vi "M4_DA_Std_FromBinaryFile.vi"() -> ()   [LabVIEW 2020]
uses:
  spcm_library/spcm_gui_common.llb/element_device.ctl
  spcm_library/spcm_gui_m4i.llb/element_m4i_ao_channel.ctl
  spcm_library/spcm_gui_m4i.llb/element_m4i_ao_trigger.ctl
  spcm_library/spcm_gui_m4i.llb/element_m4i_clock.ctl
  spcm_library/spcm_gui_m4i.llb/element_m4i_multi_purpose_io.ctl
  spcm_library/spcm_gui_common.llb/element_mode_out.ctl
  spcm_library/spcm_gui_common.llb/element_states_replay.ctl
panel:
  in  "Mode Setup":T1={"Mode"=1, "Mem"=4096, "Seg"=1024, "Loop"=0} {"Mode" items=["Singleshot", "Continuous", "Single Restart", "Multiple Replay", "Gated Replay"]; "Loop" step=1; "Mem" min=8 step=4; "Seg" min=8 step=4}
  in  "Multi Purpose IO Lines":T2={"X0 Mode"=0, "ASync Write"=8, "X1 Mode"=0, "X2 Mode"=0} {"X2 Mode" items=["Disable", "Asynchronous In", "Asynchronous Out", "Digital Input (A/D only)", "Digital Output (D/A only)", "Trigger Out", "Digital Input 2Bit (A/D only)", "Show Run State", "Show Arm State", "Ref Clock Out", "Output Marker (D/A only)", "System Clock Out"]; "X1 Mode" items=["Disable", "Asynchronous In", "Asynchronous Out", "Digital Input (A/D only)", "Digital Output (D/A only)", "Trigger Out", "Digital Input 2Bit (A/D only)", "Show Run State", "Show Arm State", "Ref Clock Out", "Output Marker (D/A only)", "System Clock Out"]; "ASync Write" min=8 step=4; "X0 Mode" items=["Disable", "Asynchronous In", "Asynchronous Out", "Digital Input (A/D only)", "Digital Output (D/A only)", "Trigger Out", "Digital Input 2Bit (A/D only)", "Show Run State", "Show Arm State", "Ref Clock Out", "Output Marker (D/A only)", "System Clock Out"]}
  in  "Clock Settings":T3={"Clock Mode"=0, "Sampling Rate (MHz)"=1250.0, "Reference Clock (MHz)"=1000.0, "Clock Output"=FALSE} {"Clock Mode" items=["Internal Clock Quartz", "External Clock (Reference Clock)", "Quartz 2 with PLL (Optional)"]; "Reference Clock (MHz)" min=10.0 max=125000.0; "Sampling Rate (MHz)" min=1.0 max=200000.0}
  in  "Reload data":bool
  out "Data Transfer Progress":i32(slide)=6 scale=0.0..100.0 scale format="%.0f %%"
  out "Replay Started":bool
  out "Data Transferred":bool
  in  "Start Data Transfer":bool
  in  "Ch3":string="waveforms\\rectangle.bin"
  in  "Ch2 File":string="waveforms\\sine.bin"
  in  "Ch1 File":string="waveforms\\Sin96.bin"
  in  "Ch0 File":string="waveforms\\Sin95.bin"
  out "Status":string="Stopped"
  in  "Trigger Settings":T4 {"Secondary Ext. Trigger" items=["None", "Pos. Edge", "Neg. Edge", "Any Edge", "High Level", "Low Level"]; "AC Coupling" items=["DC Coupling", "AC Coupling"]; "Main Ext. Trigger" items=["None", "Pos. Edge", "Neg. Edge", "Any Edge", "Pos. Rearm", "Neg. Rearm", "Enter Window", "Leave Window", "High Level", "Low Level", "In Win", "Out Win", ""]; "Trigger Source" items=["Software Trigger", "Main External Trigger", "Secondary External Trigger"]; "Trigger Delay (Samples)" max=65535 step=1}
  in  "Stop Level":cluster{"Stoplevel":u16}={"Stoplevel"=4} {"Stoplevel" items=["Tristate", "Low Level", "High Level", "Hold Last Sample", "Zero"]}
  in  "Output Channel 3":T5={"Enable"=FALSE, "Output Mode"=0, "Gain"=2000, "Offset"=0, "Filter"=0} {"Output Mode" items=["Single", "Double", "Differential"]}
  in  "Output Channel 2":T5={"Enable"=TRUE, "Output Mode"=0, "Gain"=2000, "Offset"=0, "Filter"=0} {"Output Mode" items=["Single", "Double", "Differential"]}
  in  "Output Channel 1":T5={"Enable"=FALSE, "Output Mode"=0, "Gain"=550, "Offset"=0, "Filter"=0} {"Output Mode" items=["Single", "Double", "Differential"]}
  in  "Output Channel 0":T5={"Enable"=TRUE, "Output Mode"=0, "Gain"=550, "Offset"=0, "Filter"=0} {"Output Mode" items=["Single", "Double", "Differential"]}
  in  "Singleshot Button":bool
  out "Write Setup":bool
  in  "Quit Button":bool
  in  "Force Trigger Button":bool
  in  "Stop Button":bool
  out "Device Infos":T6={"Device Name"="M4i.6622-Exp", "Serial Number"=66.0, "Mem (MB)"=4096.0}
  in  "Device":T7 {"Device" items=["Card", "digitizerNETBOX"]}
  # "Ch1"
  # "Ch0"
  # "Ch3"
  # "Ch2"
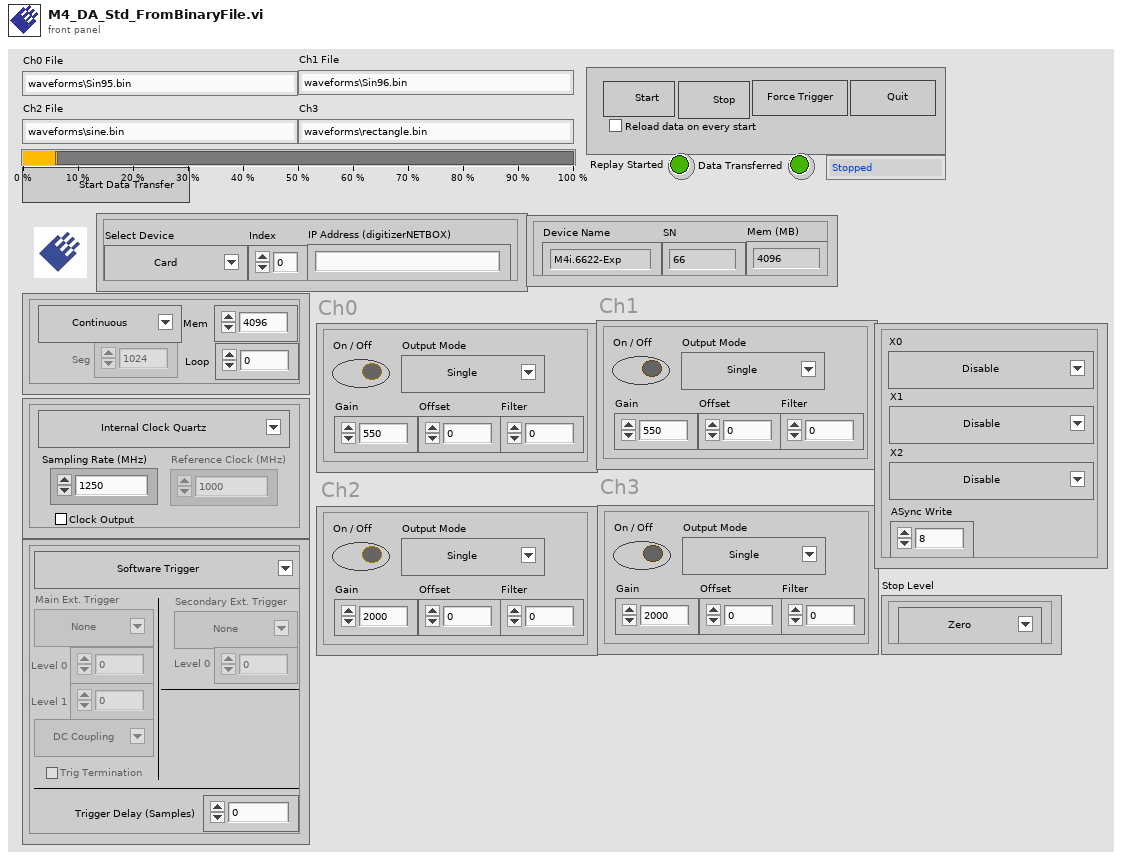
[diagram p1: front panel]
types:
  T1 = typedef "element_mode_out.ctl" = cluster{"Mode":u16, "Mem":u32, "Seg":u32, "Loop":u32}
  T2 = typedef "element_m4i_multi_purpose_io.ctl" = cluster{"X0 Mode":u16, "ASync Write":u32, "X1 Mode":u16, "X2 Mode":u16}
  T3 = typedef "element_m4i_clock.ctl" = cluster{"Clock Mode":u16, "Sampling Rate (MHz)":dbl, "Reference Clock (MHz)":dbl, "Clock Output":bool}
  T4 = typedef "element_m4i_ao_trigger.ctl" = cluster{"Trigger Source":u16, "Main Ext. Trigger":u16, "Level 0 Ext":i32, "Level 1 Ext":i32, "AC Coupling":u16, "Ext Trig Term":bool, "Secondary Ext. Trigger":u16, "Level 0 Ext1":i32, "Trigger Delay (Samples)":u32}
  T5 = typedef "element_m4i_ao_channel.ctl" = cluster{"Enable":bool, "Output Mode":u16, "Gain":i32, "Offset":i32, "Filter":i32}
  T6 = cluster{"Device Name":string, "Serial Number":dbl, "Mem (MB)":dbl}
  T7 = typedef "element_device.ctl" = cluster{"Index":dbl, "IP Address":string, "Device":u16}
  T8 = typedef "element_states_replay.ctl" = enum16{"Idle", "Init", "Write Setup", "Write Data", "Start", "Replay", "Stop", "Quit"}
  T9 = cluster{"Card Type":i32, "Inst Mem (high part)":i32, "Inst Mem (low part)":i32, "Serial Number":i32, "Function Type":i32, "Installed Features":i32, "Base Card Version":i32, "Module Version":i32, "Extension Version":i32, "Production Date":i32, "Max Sampling Rate":i32, "Max Channels":i32, "Demo Card":i32}
  T10 = cluster{"Card Name":string, "SN":i32, "Mem (MB)":i32}
  T11 = cluster{"AO Channels":i32, "Bit Resolution":i32, "AO Gain":i32, "AO Filter":i32, "AO Offset":i32}
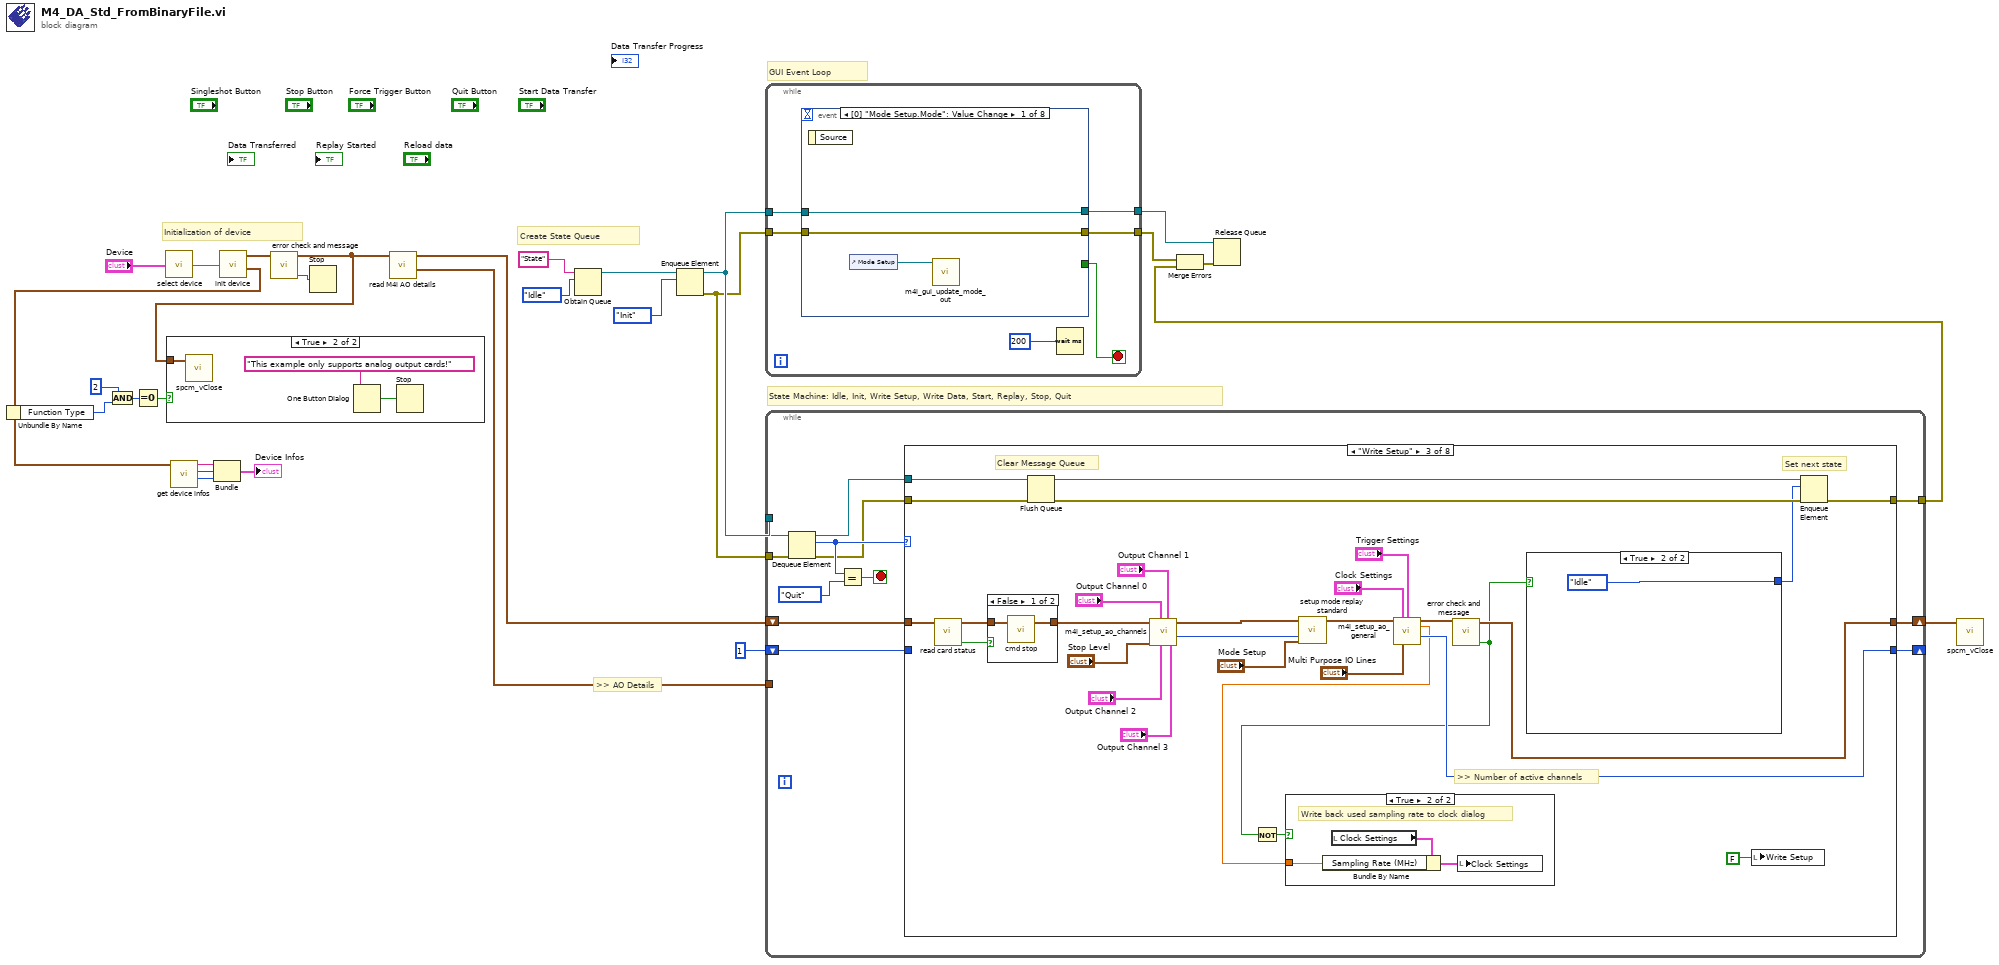
[diagram p0: block diagram]
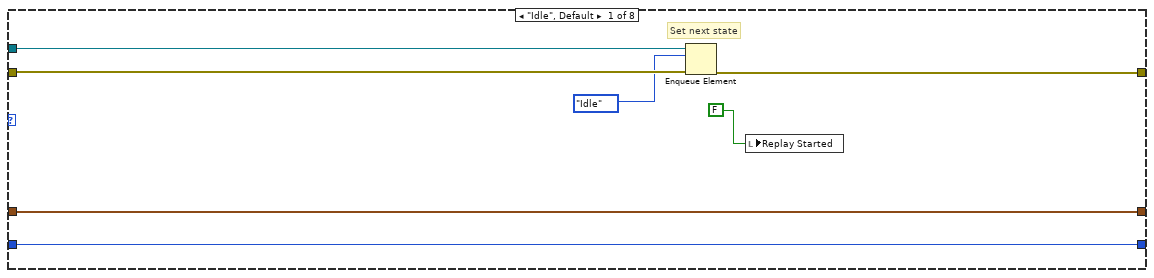
[diagram p3: hidden frame]
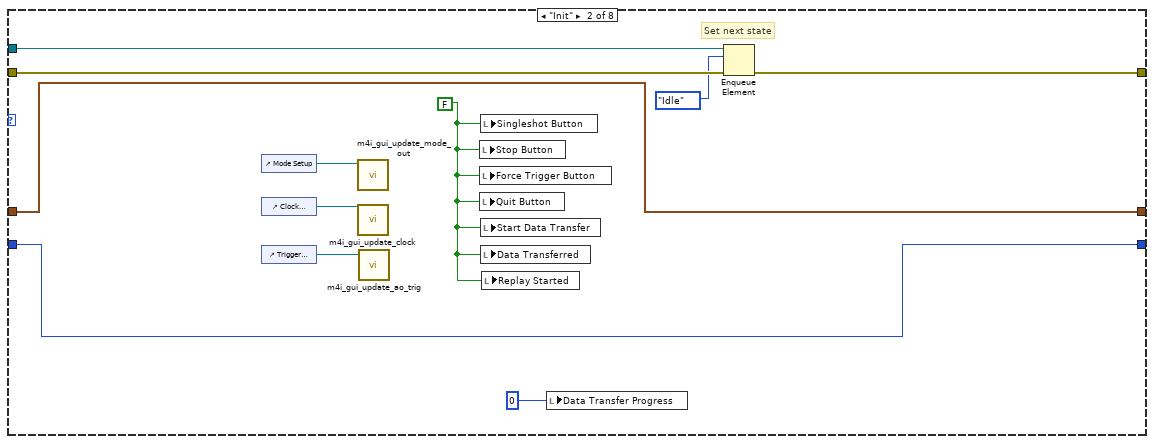
[diagram p4: hidden frame]
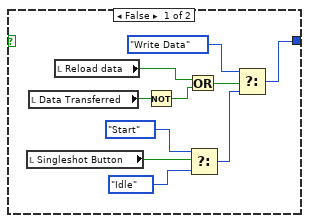
[diagram p7: hidden frame]
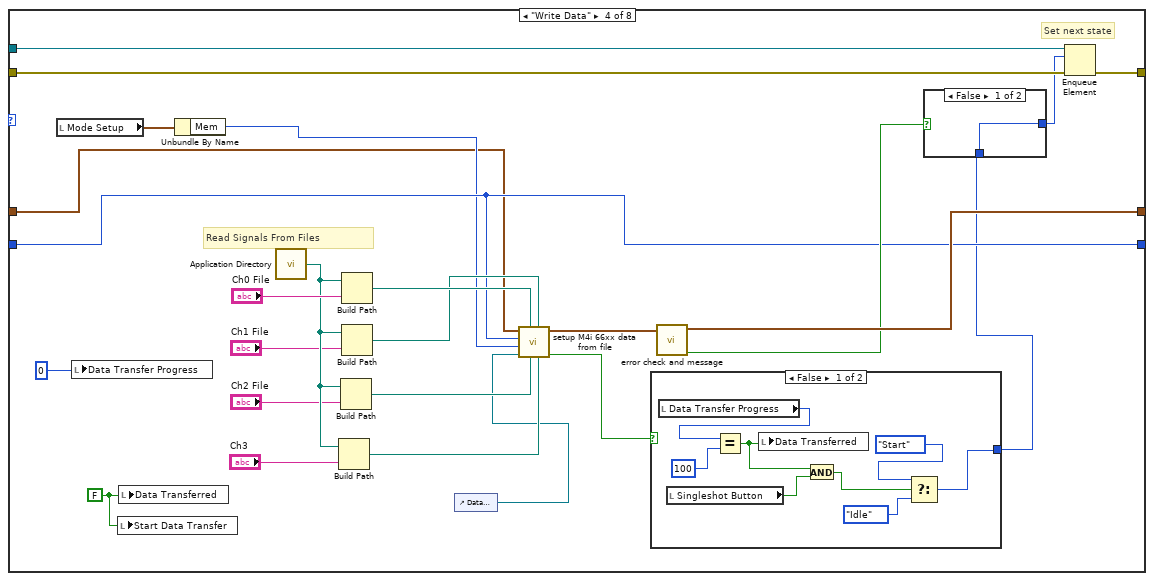
[diagram p8: hidden frame]
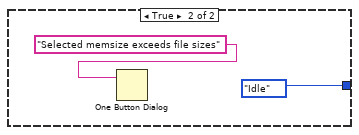
[diagram p9: hidden frame]
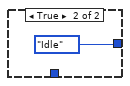
[diagram p10: hidden frame]
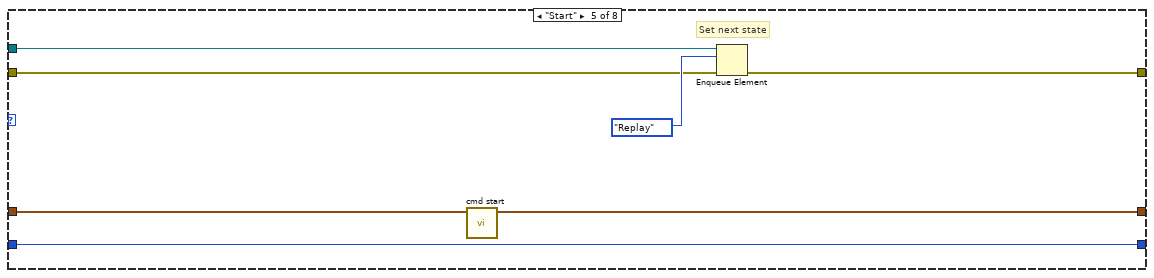
[diagram p11: hidden frame]
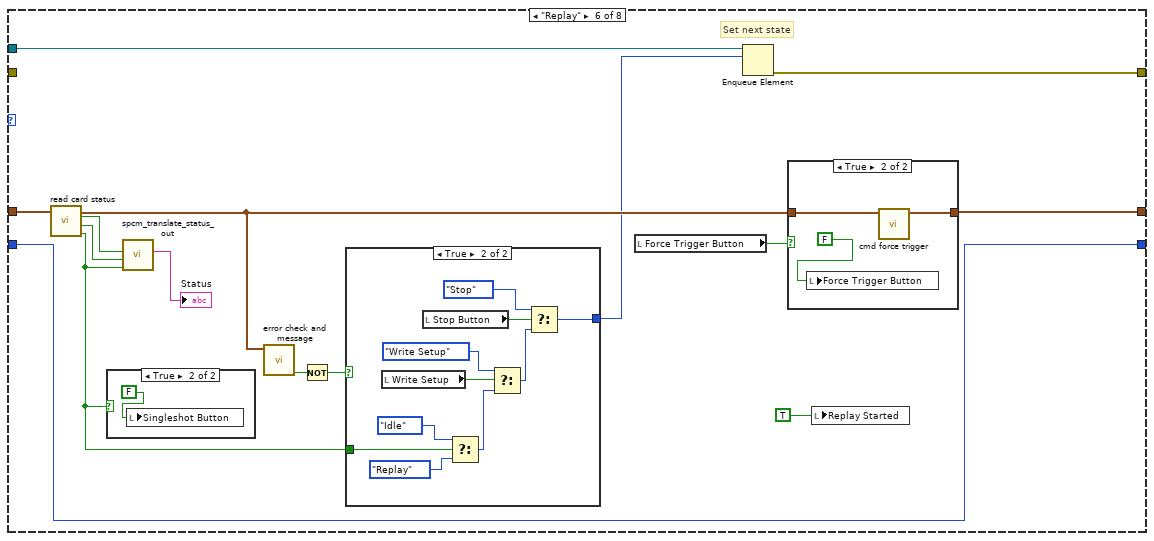
[diagram p12: hidden frame]
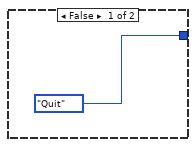
[diagram p14: hidden frame]
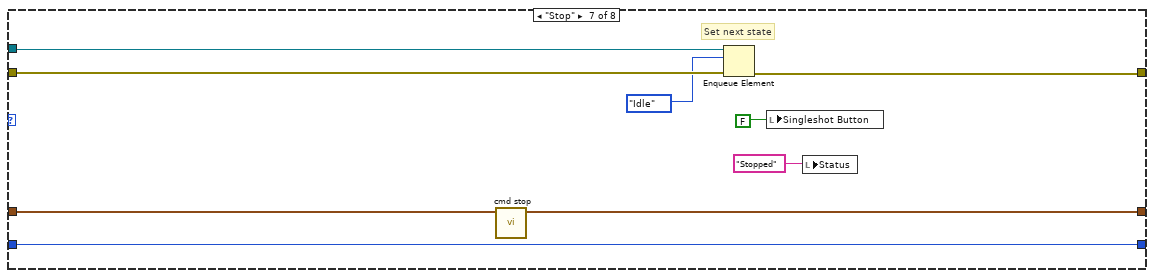
[diagram p16: hidden frame]
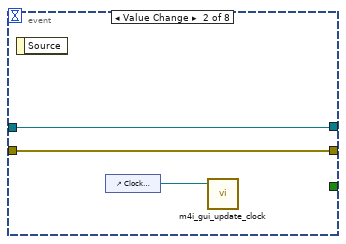
[diagram p18: hidden frame]
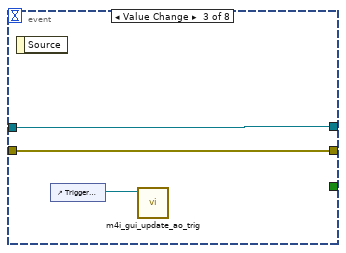
[diagram p19: hidden frame]
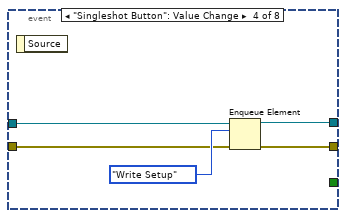
[diagram p20: hidden frame]
diagram:
  # ">> AO Details"
  # "Initialization of device"
  # "Create State Queue"
  # "State Machine: Idle, Init, Write Setup, Write Data, Start, Replay, Stop, Quit"
  # "GUI Event Loop"
  n1 = call "select device.vi"("Device"="Device") -> ("device string"=w28:string)  [unwired: 4 in]
  n2 = call "init device.vi"("Device String"=w28) -> ("Card Info Out"=w27:cluster{"Card Handle":u64, "Error Code":u32}, "Card Information"=w11:T9)  [unwired: 4 in]
  n3 = Unbundle By Name(w11) -> ("Function Type"=w15:i32)
  n4 = And(x=2, y=w15) -> (x .and. y?=w14:i32)
  n5 = Equal To 0?(x=w14) -> (x = 0?=w12:bool)
  n6 = call "get device infos.vi"("Card Information"=w11) -> ("Mem (MB)"=w19:i32, "SN"=w18:i32, "Card Name"=w17:string)  [unwired: 8 in]
  n7 = Bundle("Card Name"=w17, "SN"=w18, "Mem (MB)"=w19) -> (→"Device Infos":T10)  [unwired: 1 in]
  n8 = call "error check and message.vi"("Card Info In"=w27) -> ("Error occurred"=w26:bool, "Card Info Out"=w4:cluster{"Card Handle":u64, "Error Code":u32})  [unwired: 4 in, 1 out]
  n9 = case shown="True" w12 {
    tunnel: w4 -> [_ w29]
    frame False {
    }
    frame True {
      n10 = call "spcm_vClose.vi"("Card Info In"=w29) -> ()  [unwired: 7 in]
      n11 = One Button Dialog(message="This example only supports analog output cards!") -> (true=w30:bool)  [unwired: 1 in]
      n12 = Stop(stop? (T)=w30) -> ()
    }
  }
  n13 = Stop(stop? (T)=w26) -> ()
  n14 = call "read M4i AO details.vi"("Card Info In"=w4) -> ("AO Details"=w3:T11, "Card Info Out"=w2:cluster{"Card Handle":u64, "Error Code":u32})  [unwired: 5 in]
  n15 = Obtain Queue(name (unnamed)="State", element data type=element_states_replay."Idle") -> (queue out=w23:refnum<queue>)  [unwired: 3 in, 2 out]
  n16 = Enqueue Element(queue=w23, element=element_states_replay."Init") -> (queue out=w24:refnum<queue>, error out=w6:errorcluster)  [unwired: 2 in, 1 out]
  n17 = while {
    tunnel: w24 -> [w35]
    tunnel: [w36] -> w7
    tunnel: [w32] -> w10
    tunnel: w6 -> [w33]
    stop <- w34 stop-if-true
    n18 = event shown="[0] \"Mode Setup.Mode\": Value Change" {
      selector: _ -> [_ _ _ _ _ _ _ _]
      dyn-events: _ -> [_ _ _ _ _ _ _ _]
      timeout: _ -> [_ _ _ _ _ _ _ _]
      tunnel: [_ _ _ _ _ _ TRUE _] -> w34
      tunnel: [w40 w43 w46 w51 w56 w62 w67 w71] -> w36
      tunnel: w35 -> [w40 w43 w46 w48 w55 w61 w68 w71]
      tunnel: [w39 w42 w45 w50 w53 w59 w65 w70] -> w32
      tunnel: w33 -> [w39 w42 w45 w47 w54 w60 w64 w70]
      event Value Change {
        n19 = event-data ("Ereignisdatenknoten")() -> ()  [unwired: 1 in, 1 out]
        n20 = control-ref of="Mode Setup"() -> (w38:refnum<vi>)
        n21 = call "m4i_gui_update_mode_out.vi"("Cluster Referenz"=w38) -> ()  [unwired: 11 in]
      }
      event Value Change {
        n22 = event-data() -> ()  [unwired: 1 in, 1 out]
        n23 = control-ref of="Clock Settings"() -> (w41:refnum<vi>)
        n24 = call "m4i_gui_update_clock.vi"("Cluster Reference"=w41) -> ()  [unwired: 11 in]
      }
      event Value Change {
        n25 = event-data() -> ()  [unwired: 1 in, 1 out]
        n26 = control-ref of="Trigger Settings"() -> (w44:refnum<vi>)
        n27 = call "m4i_gui_update_ao_trig.vi"("Cluster Referenz"=w44) -> ()  [unwired: 11 in]
      }
      event "Singleshot Button": Value Change {
        n28 = event-data() -> ()  [unwired: 1 in, 1 out]
        n29 = Enqueue Element(queue=w48, element=element_states_replay."Write Setup", error in (no error)=w47) -> (queue out=w51:refnum<queue>, error out=w50:errorcluster)  [unwired: 1 in, 1 out]
      }
      event "Stop Button": Value Change {
        n30 = event-data() -> ()  [unwired: 1 in, 1 out]
        n31 = Enqueue Element(queue=w55, element=element_states_replay."Stop", error in (no error)=w54) -> (queue out=w56:refnum<queue>, error out=w53:errorcluster)  [unwired: 1 in, 1 out]
      }
      event "Start Data Transfer": Value Change {
        n32 = event-data() -> ()  [unwired: 1 in, 1 out]
        n33 = local write "Data Transferred"(FALSE) -> ()
        n34 = Enqueue Element(queue=w61, element=element_states_replay."Write Setup", error in (no error)=w60) -> (queue out=w62:refnum<queue>, error out=w59:errorcluster)  [unwired: 1 in, 1 out]
      }
      event "Quit Button": Value Change {
        n35 = event-data() -> ()  [unwired: 1 in, 1 out]
        n36 = Enqueue Element(queue=w68, element=element_states_replay."Quit", error in (no error)=w64) -> (queue out=w67:refnum<queue>, error out=w65:errorcluster)  [unwired: 1 in, 1 out]
      }
      event Value Change {
        n37 = event-data() -> ()  [unwired: 1 in, 1 out]
        "Write Setup" <- TRUE
      }
    }
    n38 = Wait (ms)(milliseconds to wait=200) -> ()  [unwired: 1 out]
  }
  n39 = while {
    tunnel: w24 -> [w83]
    shift-right: [w81] -> w22
    shift-left: w2 -> [w82]
    shift-right: [w76] -> _
    shift-left: 1 -> [w77]
    tunnel: [w75] -> w9
    tunnel: w6 -> [w74]
    tunnel: w3 -> [_]
    stop <- w79 stop-if-true
    n40 = Dequeue Element(queue=w83, error in (no error)=w74) -> (queue out=w78:refnum<queue>, element=w80:T8, error out=w73:errorcluster)  [unwired: 1 in, 1 out]
    n41 = Equal?(x=w80, y=element_states_replay."Quit") -> (x = y?=w79:bool)
    n42 = case shown="\"Write Setup\"" w80 {
      tunnel: w82 -> [w90 w98 w115 w154 w187 w203 w227 w233]
      tunnel: [w90 w98 w111 w168 w186 w196 w226 w233] -> w81
      tunnel: w78 -> [w85 w101 w117 w170 w185 w199 w230 _]
      tunnel: w77 -> [w89 w97 _ w156 w190 w194 w225 w232]
      tunnel: [w89 w97 w125 w156 w190 w194 w225 w232] -> w76
      tunnel: [w87 w100 w128 w169 w189 w197 w228 w231] -> w75
      tunnel: w73 -> [w88 w99 w129 w171 w184 _ w229 w231]
      frame "Idle", Default {
        # "Set next state"
        n43 = Enqueue Element(queue=w85, element=element_states_replay."Idle", error in (no error)=w88) -> (error out=w87:errorcluster)  [unwired: 1 in, 2 out]
        n44 = local write "Replay Started"(FALSE) -> ()
      }
      frame "Init" {
        w94 = FALSE
        # "Set next state"
        n45 = control-ref of="Mode Setup"() -> (w91:refnum<vi>)
        n46 = control-ref of="Clock Settings"() -> (w92:refnum<vi>)
        n47 = control-ref of="Trigger Settings"() -> (w95:refnum<vi>)
        n48 = call "m4i_gui_update_mode_out.vi"("Cluster Referenz"=w91) -> ()  [unwired: 11 in]
        n49 = call "m4i_gui_update_clock.vi"("Cluster Reference"=w92) -> ()  [unwired: 11 in]
        n50 = call "m4i_gui_update_ao_trig.vi"("Cluster Referenz"=w95) -> ()  [unwired: 11 in]
        n51 = local write "Stop Button"(w94) -> ()
        n52 = local write "Force Trigger Button"(w94) -> ()
        n53 = local write "Quit Button"(w94) -> ()
        n54 = local write "Singleshot Button"(w94) -> ()
        n55 = local write "Start Data Transfer"(w94) -> ()
        n56 = local write "Data Transferred"(w94) -> ()
        n57 = local write "Replay Started"(w94) -> ()
        n58 = local write "Data Transfer Progress"(0) -> ()
        n59 = Enqueue Element(queue=w101, element=element_states_replay."Idle", error in (no error)=w99) -> (error out=w100:errorcluster)  [unwired: 1 in, 2 out]
      }
      frame "Write Setup" {
        # "Set next state"
        # "Clear Message Queue"
        # ">> Number of active channels"
        n60 = call "read card status.vi"("Card Info In"=w115) -> ("Card ready"=w112:bool, "Card Info Out"=w114:cluster{"Card Handle":u64, "Error Code":u32})  [unwired: 3 in, 2 out]
        n61 = case shown="False" w112 {
          tunnel: w114 -> [w134 w135]
          tunnel: [w133 w135] -> w113
          frame False {
            n62 = call "cmd stop.vi"("Card Info In"=w134) -> ("Card Info Out"=w133:cluster{"Card Handle":u64, "Error Code":u32})  [unwired: 6 in]
          }
          frame True {
          }
        }
        n63 = Flush Queue(queue=w117) -> (queue out=w116:refnum<queue>)  [unwired: 1 in, 2 out]
        n64 = call "m4i_setup_ao_channels.vi"("Output Channel 3"="Output Channel 3", "Output Channel 1"="Output Channel 1", "Output Channel 2"="Output Channel 2", "Output Channel 0"="Output Channel 0", "Stop Level"="Stop Level", "Card Info In"=w113) -> ("ChMask"=w103:i32, "Card Info Out"=w104:cluster{"Card Handle":u64, "Error Code":u32})  [unwired: 3 in, 1 out]
        n65 = call "setup mode replay standard.vi"("Mode Setup"="Mode Setup", "Channel Mask Low"=w103, "Card Info In"=w104) -> ("Card Info Out"=w105:cluster{"Card Handle":u64, "Error Code":u32})  [unwired: 4 in]
        n66 = call "m4i_setup_ao_general.vi"("Card Info In"=w105, "Clock Settings"="Clock Settings", "Trigger Settings"="Trigger Settings", "Multi Purpose IO Lines"="Multi Purpose IO Lines") -> ("Card Info Out"=w118:cluster{"Card Handle":u64, "Error Code":u32}, "Used Sampling Rate (MS)"=w109:dbl, "Channel Count"=w125:i32)  [unwired: 7 in, 2 out]
        n67 = call "error check and message.vi"("Card Info In"=w118) -> ("Error occurred"=w106:bool, "Card Info Out"=w111:cluster{"Card Handle":u64, "Error Code":u32})  [unwired: 4 in, 1 out]
        n68 = Not(x=w106) -> (.not. x?=w107:bool)
        n69 = case shown="True" w107 {
          tunnel: w109 -> [_ w130]
          frame False {
          }
          frame True {
            # "Write back used sampling rate to clock dialog"
            n70 = local read "Clock Settings"() -> (w132:T3)
            n71 = Bundle By Name(cluster=w132, "Sampling Rate (MHz)"=w130) -> (w131:T3)
            n72 = local write "Clock Settings"(w131) -> ()
          }
        }
        n73 = case shown="True" w106 {
          tunnel: [w140 element_states_replay."Idle"] -> w127
          frame False {
            n74 = local read "Singleshot Button"() -> (w137:bool)
            n75 = local read "Data Transferred"() -> (w141:bool)
            n76 = local read "Reload data"() -> (w143:bool)
            n77 = Not(x=w141) -> (.not. x?=w142:bool)
            n78 = Or(x=w143, y=w142) -> (x .or. y?=w144:bool)
            n79 = Select(t=element_states_replay."Start", s=w137, f=element_states_replay."Idle") -> (s? t:f=w136:T8)
            n80 = Select(t=element_states_replay."Write Data", s=w144, f=w136) -> (s? t:f=w140:T8)
          }
          frame True {
          }
        }
        n81 = local write "Write Setup"(FALSE) -> ()
        n82 = Enqueue Element(queue=w116, element=w127, error in (no error)=w129) -> (error out=w128:errorcluster)  [unwired: 1 in, 2 out]
      }
      frame "Write Data" {
        w148 = FALSE
        # "Read Signals From Files"
        # "Set next state"
        n83 = local read "Mode Setup"() -> (w147:T1)
        n84 = local write "Data Transfer Progress"(0) -> ()
        n85 = local write "Start Data Transfer"(w148) -> ()
        n86 = local write "Data Transferred"(w148) -> ()
        n87 = Unbundle By Name(w147) -> ("Mem"=w155:u32)
        n88 = call <vilib>:"Application Directory.vi"() -> ("Application Directory"=w164:path)
        n89 = Build Path(base path=w164, name or relative path="Ch3") -> (appended path=w157:path)
        n90 = Build Path(base path=w164, name or relative path="Ch2 File") -> (appended path=w158:path)
        n91 = Build Path(base path=w164, name or relative path="Ch0 File") -> (appended path=w160:path)
        n92 = Build Path(base path=w164, name or relative path="Ch1 File") -> (appended path=w159:path)
        n93 = control-ref of="Data Transfer Progress"() -> (w152:refnum<vi>)
        n94 = call "setup M4i 66xx data from file.vi"("File Path Ch3"=w157, "File Path Ch1"=w159, "File Path Ch2"=w158, "File Path Ch0"=w160, "Ref Progress"=w152, "Length (Samples per channel)"=w155, "Number of channels"=w156, "Card Info In"=w154) -> ("Length exceeds file size"=w151:bool, "Card Info Out"=w153:cluster{"Card Handle":u64, "Error Code":u32})  [unwired: 2 in]
        n95 = case shown="False" w151 {
          tunnel: [w175 element_states_replay."Idle"] -> w150
          frame False {
            n96 = local read "Data Transfer Progress"() -> (w178:i32)
            n97 = local read "Singleshot Button"() -> (w176:bool)
            n98 = Equal?(x=w178, y=100) -> (x = y?=w177:bool)
            n99 = local write "Data Transferred"(w177) -> ()
            n100 = And(x=w177, y=w176) -> (x .and. y?=w174:bool)
            n101 = Select(t=element_states_replay."Start", s=w174, f=element_states_replay."Idle") -> (s? t:f=w175:T8)
          }
          frame True {
            n102 = One Button Dialog(message="Selected memsize exceeds file sizes") -> ()  [unwired: 1 in, 1 out]
          }
        }
        n103 = call "error check and message.vi"("Card Info In"=w153) -> ("Error occurred"=w167:bool, "Card Info Out"=w168:cluster{"Card Handle":u64, "Error Code":u32})  [unwired: 4 in, 1 out]
        n104 = case shown="False" w167 {
          tunnel: [w182 element_states_replay."Idle"] -> w166
          tunnel: w150 -> [w182 _]
          frame False {
          }
          frame True {
          }
        }
        n105 = Enqueue Element(queue=w170, element=w166, error in (no error)=w171) -> (error out=w169:errorcluster)  [unwired: 1 in, 2 out]
      }
      frame "Start" {
        # "Set next state"
        n106 = call "cmd start.vi"("Card Info In"=w187) -> ("Card Info Out"=w186:cluster{"Card Handle":u64, "Error Code":u32})  [unwired: 6 in]
        n107 = Enqueue Element(queue=w185, element=element_states_replay."Replay", error in (no error)=w184) -> (error out=w189:errorcluster)  [unwired: 1 in, 2 out]
      }
      frame "Replay" {
        # "Set next state"
        n108 = call "read card status.vi"("Card Info In"=w203) -> ("Card ready"=w191:bool, "Trigger detected"=w205:bool, "Pretrigger full"=w204:bool, "Card Info Out"=w202:cluster{"Card Handle":u64, "Error Code":u32})  [unwired: 3 in]
        n109 = case shown="True" w191 {
          frame False {
          }
          frame True {
            n110 = local write "Singleshot Button"(FALSE) -> ()
          }
        }
        n111 = call "spcm_translate_status_out.vi"("Ready"=w191, "Trigger"=w205, "Pretrigger"=w204) -> ("Text"=→"Status":string)  [unwired: 4 in]
        n112 = call "error check and message.vi"("Card Info In"=w202) -> ("Error occurred"=w201:bool)  [unwired: 4 in, 2 out]
        n113 = Not(x=w201) -> (.not. x?=w200:bool)
        n114 = case shown="True" w200 {
          tunnel: [element_states_replay."Quit" w212] -> w198
          tunnel: w191 -> [_ w217]
          frame False {
          }
          frame True {
            n115 = local read "Write Setup"() -> (w211:bool)
            n116 = local read "Stop Button"() -> (w214:bool)
            n117 = Select(t=element_states_replay."Idle", s=w217, f=element_states_replay."Replay") -> (s? t:f=w209:T8)
            n118 = Select(t=element_states_replay."Write Setup", s=w211, f=w209) -> (s? t:f=w208:T8)
            n119 = Select(t=element_states_replay."Stop", s=w214, f=w208) -> (s? t:f=w212:T8)
          }
        }
        n120 = local read "Force Trigger Button"() -> (w193:bool)
        n121 = Enqueue Element(queue=w199, element=w198) -> (error out=w197:errorcluster)  [unwired: 2 in, 2 out]
        n122 = case shown="True" w193 {
          tunnel: w202 -> [w218 w219]
          tunnel: [w218 w221] -> w196
          frame False {
          }
          frame True {
            n123 = local write "Force Trigger Button"(FALSE) -> ()
            n124 = call "cmd force trigger.vi"("Card Info In"=w219) -> ("Card Info Out"=w221:cluster{"Card Handle":u64, "Error Code":u32})  [unwired: 6 in]
          }
        }
        n125 = local write "Replay Started"(TRUE) -> ()
      }
      frame "Stop" {
        # "Set next state"
        n126 = call "cmd stop.vi"("Card Info In"=w227) -> ("Card Info Out"=w226:cluster{"Card Handle":u64, "Error Code":u32})  [unwired: 6 in]
        n127 = Enqueue Element(queue=w230, element=element_states_replay."Idle", error in (no error)=w229) -> (error out=w228:errorcluster)  [unwired: 1 in, 2 out]
        n128 = local write "Singleshot Button"(FALSE) -> ()
        n129 = local write "Status"("Stopped") -> ()
      }
      frame "Quit" {
      }
    }
  }
  n130 = Merge Errors(w10, w9) -> (w8:errorcluster)
  n131 = Release Queue(queue=w7, error in (no error)=w8) -> ()  [unwired: 1 in, 3 out]
  n132 = call "spcm_vClose.vi"("Card Info In"=w22) -> ()  [unwired: 7 in]
